vi "take piece from cube.vi"(1 "y":dbl, 2 "level":i32) -> ()   [LabVIEW 2018]
uses:
  vision/vision info 2.vi
panel:
  in  "speed":dbl
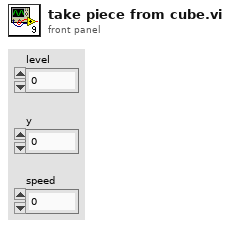
[diagram p1: front panel]
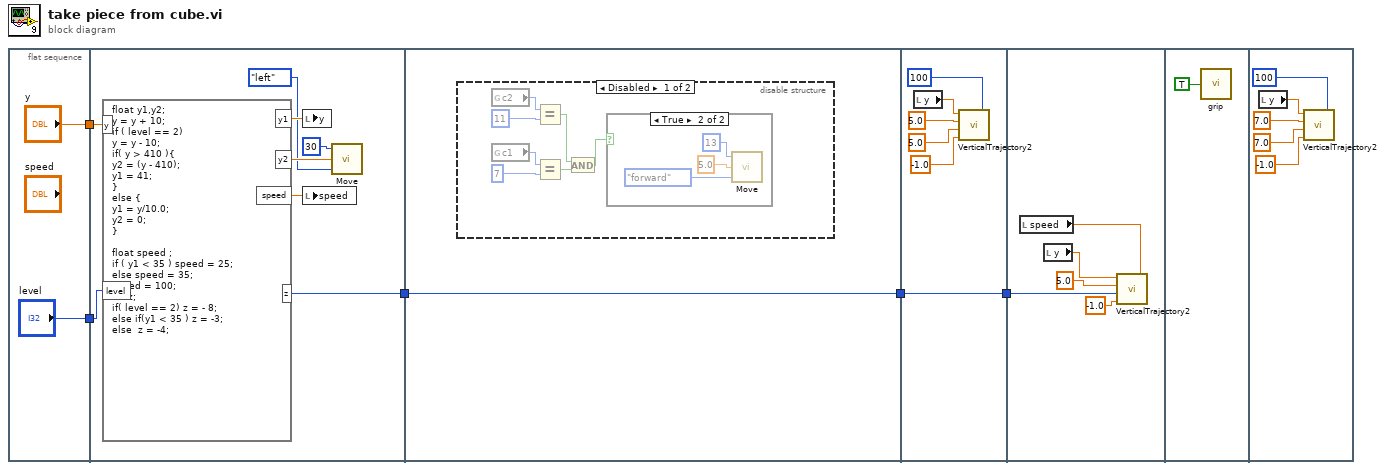
[diagram p0: block diagram]
diagram:
  n1 = flat-sequence {
    tunnel: ["y"] -> w5
    tunnel: ["level"] -> w1
    tunnel: w5 -> [w10]
    tunnel: [w9] -> w3
    tunnel: w1 -> [w8]
    tunnel: w3 -> [w16]
    tunnel: [w16] -> w2
    tunnel: [w27] -> w4
    tunnel: w2 -> [w27]
    tunnel: w4 -> [w33]
    frame #0 {
    }
    frame #1 {
      n2 = formula code="float y1,y2;\ny = y + 10;\nif ( level == 2) \ny = y - 10;\nif( y > 410 ){\ny2 = (y - 410);\ny1 = 41;\n}\nelse {\ny1 = y/10.0;\ny2 = 0;\n}\n\nfloat speed ;\nif ( y1 < 35 ) speed = 25;\nelse speed = 35;\nspeed = 100;\nint z;\nif( level == 2) z = - 8;\nelse if(y1 < 35 ) z = -3;\nelse  z = -4;"("y"=w10, "level"=w8) -> ("y1"=w14:dbl, "y2"=w13:dbl, "speed"=w15:dbl, "z"=w9:i32)
      n3 = local write "y"(w14) -> ()
      n4 = local write "speed"(w15) -> ()
      n5 = call "Move.vi"("Enum"=enum16{"forward", "backward", "left", "right"}."left", "distance"=w13, "speed"=30) -> ()  [unwired: 1 in]
    }
    frame #2 {
      n6 = disable-structure shown="Disabled" {
        frame Disabled {
          n7 = global read "vision info 2.vi" "c2"() -> (w23:i8)
          n8 = global read "vision info 2.vi" "c1"() -> (w22:i8)
          n9 = Equal?(x=w23, y=i8 11) -> (x = y?=w18:bool)
          n10 = Equal?(x=w22, y=i8 7) -> (x = y?=w17:bool)
          n11 = And(x=w18, y=w17) -> (x .and. y?=w19:bool)
          n12 = case shown="True" w19 {
            frame False {
            }
            frame True {
              n13 = call "Move.vi"("Enum"=enum16{"forward", "backward", "left", "right"}."forward", "distance"=5.0, "speed"=13) -> ()  [unwired: 1 in]
            }
          }
        }
        frame Enabled {
        }
      }
    }
    frame #3 {
      n14 = local read "y"() -> (w29:dbl)
      n15 = call "VerticalTrajectory2.vi"("speed 1"=100, "step"=-1.0, "z2"=5.0, "z1"=5.0, "x"=w29) -> ()  [unwired: 3 in]
    }
    frame #4 {
      n16 = local read "speed"() -> (w34:dbl)
      n17 = local read "y"() -> (w37:dbl)
      n18 = call "VerticalTrajectory2.vi"("speed 1"=w34, "step"=-1.0, "z2"=w33, "z1"=5.0, "x"=w37) -> ()  [unwired: 3 in]
    }
    frame #5 {
      n19 = call "grip.vi"("grip"=TRUE) -> ()
    }
    frame #6 {
      n20 = local read "y"() -> (w40:dbl)
      n21 = call "VerticalTrajectory2.vi"("speed 1"=100, "step"=-1.0, "z2"=7.0, "z1"=7.0, "x"=w40) -> ()  [unwired: 3 in]
    }
  }
